vi "Save Image.vi"(0 "Display State In":T2 {"ROI"."Contours"."Type" items=["No Selection", "Point", "Line", "Rectangle", "Oval", "Polygon", "Freehand Region", "Annulus", "Unused2", "Unused3", "Broken Line", "Freehand Line", "Rotated Rectangle"]}, 9 "Container State":T7, 11 "error in (no error)":errorcluster) -> (4 "Display State Out":T2 {"ROI"."Contours"."Type" items=["No Selection", "Point", "Line", "Rectangle", "Oval", "Polygon", "Freehand Region", "Annulus", "Unused2", "Unused3", "Broken Line", "Freehand Line", "Rotated Rectangle"]}, 15 "error out":errorcluster)   [LabVIEW 2009, in "POLARIS IMAQ Display.xctl"]
uses:
  POLARIS IMAQ Display.xctl
  <vilib>/_xctls/Container State.ctl
  State.ctl
  IMAQdx Cam/IMAQdx Cam.lvclass
  Properties/ImageSource.ctl
  <vilib>/vision/Image Controls.llb/IMAQ Image.ctl
  DisplaySettings.ctl
  Named ROI.ctl
  Analyze Classes/Analyze BaseClass/Analyze BaseClass.lvclass
  Palette.ctl
  <vilib>/Utility/config.llb/NI_LVConfig.lvlib
  <vilib>/_xctls/XControlSupport.lvlib
panel:
  out "Image":T1(plugin-control)
  # "Add Controls & Indicators that form the parameters of the method here. Hook them to the connector pane. Do not delete the controls & indicators that are already hooked to the connector pane.\n \nTo setup the parameters  for this method, right click on this item in the Project Tree & select \"Configure Method...\"."
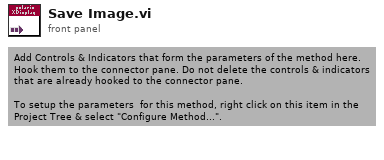
[diagram p1: front panel]
types:
  T1 = typedef "IMAQ Image.ctl" = refnum<image>
  T2 = typedef "POLARIS IMAQ Display.xctl/State.ctl" = cluster{"ImageSource":T3, "IMAQdx Cam":refnum<class "IMAQdx Cam.lvclass">, "WorkDir":path, "Image Name Prefix":string, "ROI":T4, "BG Image":T1, "Display Image":T1, "Display settings":T5, "Mask image":T1, "ConfigDir":path, "Display ref":refnum<vi>, "Saved ROIs":T6[], "Selected ROI":string, "Analyze Objects":refnum<class "Analyze BaseClass.lvclass">[], "Analysis Params":variant, "Analysis Results":variant, "Overlays?":bool[], "Ref Palette type":refnum<vi>, "Time in Filename?":bool, "Save Report?":bool, "Appl Params":variant, "Show ZoomBtn?":bool}
  T3 = typedef "POLARIS IMAQ Display.xctl/ImageSource.ctl" = enum16{"Camera", "File"}
  T4 = typedef "ROI Descriptor" = cluster{"Global Rectangle":i32[], "Contours":cluster{"ID":enum32{"External", "Internal"}, "Type":u32, "Coordinates":i32[]}[]}
  T5 = typedef "POLARIS IMAQ Display.xctl/DisplaySettings.ctl" = cluster{"Min. Thresh.":sgl, "X":dbl, "Y":dbl, "ShowLineout":bool, "ScaleParts":i32, "ShowLegende":bool, "Target Cross":bool, "Centroid Cross":bool, "Target color":u32, "Centroid color":u32, "calibr. mm/px":sgl}
  T6 = typedef "POLARIS IMAQ Display.xctl/Named ROI.ctl" = cluster{"ROI":cluster{"Global Rectangle":i32[], "Contours":cluster{"Contour Type":u32, "ROI Type":u32, "Points":i32[]}[]}, "Name":string}
  T7 = typedef "XControlSupport.lvlib/Container State.ctl" = cluster{"Indicator?":bool, "Run Mode?":bool, " Refnum":refnum<vi>}
  T8 = typedef "IMAQdx.ctl" = refnum<k21>
  T9 = cluster{"Global Rectangle":i32[], "Contours":cluster{"Contour Type":u32, "ROI Type":u32, "Points":i32[]}[]}
  T10 = typedef "NI_LVConfig.lvlib/Config Data RefNum.ctl" = refnum<k1>
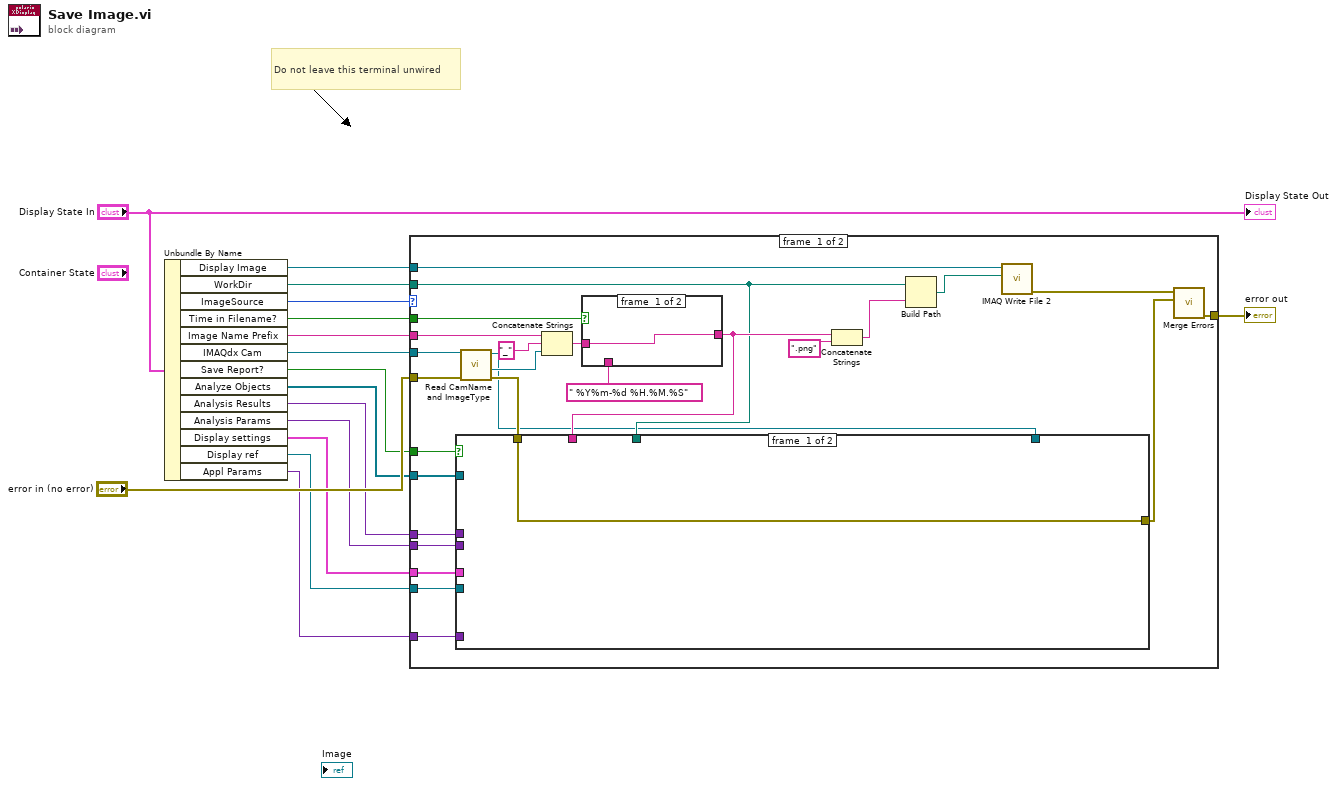
[diagram p0: block diagram]
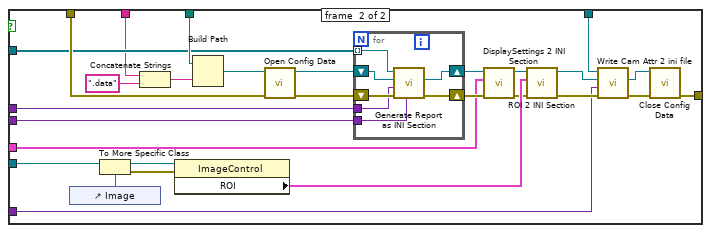
[diagram p2: hidden frame]
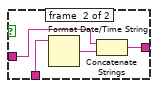
[diagram p3: hidden frame]
diagram:
  # "Do not leave this terminal unwired"
  n1 = Unbundle By Name("Display State In") -> ("Display Image"=w4:T1, "WorkDir"=w12:path, "ImageSource"=w11:T3, "Time in Filename?"=w2:bool, "Image Name Prefix"=w15:string, "IMAQdx Cam"=w16:refnum<class "IMAQdx Cam.lvclass">, "Save Report?"=w10:bool, "Analyze Objects"=w5:refnum<class "Analyze BaseClass.lvclass">[], "Analysis Results"=w7:variant, "Analysis Params"=w6:variant, "Display settings"=w9:T5, "Display ref"=w8:refnum<vi>, "Appl Params"=w1:variant)
  n2 = case shown="\"Camera\", Default" w11 {
    tunnel: w16 -> [w42 _]
    tunnel: w15 -> [w40 _]
    tunnel: "error in (no error)" -> [w38 w84]
    tunnel: w8 -> [w37 _]
    tunnel: w12 -> [w19 _]
    tunnel: w9 -> [w35 _]
    tunnel: w6 -> [w32 _]
    tunnel: w7 -> [w33 _]
    tunnel: w2 -> [w29 _]
    tunnel: w10 -> [w27 _]
    tunnel: w5 -> [w26 _]
    tunnel: w4 -> [w25 _]
    tunnel: [w20 w84] -> w3
    tunnel: w1 -> [w17 _]
    frame #0 {
      n3 = call-dynamic "Read CamName and ImageType.vi"("error in (no error)"=w38, "IMAQdx Cam in"=w42) -> ("error out"=w34:errorcluster, "Camera"=w39:T8, "IMAQdx Cam out"=w18:refnum<class "IMAQdx Cam.lvclass">)  [unwired: 6 in, 1 out]
      n4 = Concatenate Strings(w40, "_" ("string"), w39) -> (w30:string)
      n5 = case shown="True" w29 {
        tunnel: [w79 w81] -> w31
        tunnel: w30 -> [w79 w80]
        tunnel: " %Y%m-%d %H.%M.%S" ("time format string (%c)") -> [_ w83]
        frame #0 {
        }
        frame #1 {
          n6 = Format Date/Time String(time format string (%c)=w83) -> (date/time string=w82:string)  [unwired: 2 in]
          n7 = Concatenate Strings(w80, w82) -> (w81:string)
        }
      }
      n8 = case shown="True" w27 {
        tunnel: w37 -> [_ w71]
        tunnel: w19 -> [_ w68]
        tunnel: w35 -> [_ w50]
        tunnel: w34 -> [w43 w65]
        tunnel: [w43 w64] -> w21
        tunnel: w26 -> [_ w63]
        tunnel: w33 -> [_ w62]
        tunnel: w32 -> [_ w61]
        tunnel: w31 -> [_ w60]
        tunnel: w18 -> [_ w49]
        tunnel: w17 -> [_ w44]
        frame #0 {
        }
        frame #1 {
          n9 = control-ref of="Image"() -> (w56:refnum<vi>)
          n10 = To More Specific Class(target class=w56, reference=w71) -> (specific class reference=w70:refnum<vi>, error out=w55:errorcluster)  [unwired: 1 in]
          n11 = Concatenate Strings(w60, ".data" ("string")) -> (w67:string)
          n12 = property class="ImageControl"(reference=w70, error in=w55) -> ("ROI"=w57:T9)  [unwired: 2 out]
          n13 = Build Path(base path=w68, name or relative path=w67) -> (appended path=w66:path)
          n14 = call <vilib>:"Open Config Data.vi"("error in (no error)"=w65, "configuration file path"=w66) -> ("error out"=w59:errorcluster, "refnum"=w58:T10)  [unwired: 7 in, 1 out]
          n15 = for {
            tunnel: w63 -> [w78] mode=indexing
            shift-right: [w74] -> w54
            shift-left: w58 -> [w77]
            shift-right: [w75] -> w51
            shift-left: w59 -> [w76]
            tunnel: w62 -> [w73]
            tunnel: w61 -> [w72]
            n16 = call-dynamic "Generate Report as INI Section.vi"("Parameters"=w72, "error in (no error)"=w76, "Results"=w73, "Refnum in"=w77, "Analyze BaseClass in"=w78) -> ("error out"=w75:errorcluster, "Refnum out"=w74:T10)  [unwired: 4 in, 1 out]
          }
          n17 = call "DisplaySettings 2 INI Section.vi"("error in (no error)"=w51, "Display settings"=w50, "refnum in"=w54) -> ("error out"=w52:errorcluster, "refnum out"=w53:T10)  [unwired: 7 in]
          n18 = call "ROI 2 INI Section.vi"("error in (no error)"=w52, "ROI Descriptor"=w57, "refnum in"=w53) -> ("error out"=w48:errorcluster, "refnum out"=w47:T10)  [unwired: 7 in]
          n19 = call "Write Cam Attr 2 ini file.vi"("error in (no error)"=w48, "Appl Params"=w44, "refnum in"=w47, "IMAQdx Cam in"=w49) -> ("error out"=w45:errorcluster, "refnum out"=w46:T10)  [unwired: 4 in, 2 out]
          n20 = call <vilib>:"Close Config Data.vi"("error in (no error)"=w45, "refnum"=w46) -> ("error out"=w64:errorcluster)  [unwired: 8 in, 1 out]
        }
      }
      n21 = Concatenate Strings(w31, ".png" ("string")) -> (w24:string)
      n22 = Build Path(base path=w19, name or relative path=w24) -> (appended path=w23:path)
      n23 = call-poly "IMAQ Write File 2"("File Path"=w23, "Image"=w25) -> ("error out"=w22:errorcluster)  [unwired: 8 in, 1 out]
      n24 = call <vilib>:"Merge Errors.vi"("error in 2 (no error)"=w21, "error in 1 (no error)"=w22) -> ("error out"=w20:errorcluster)  [unwired: 5 in]
    }
    frame #1 {
      # "Was hier zu tun ist, muss man sich noch \nüberlegen."
    }
  }
  "error out" <- w3
  "Display State Out" <- "Display State In"
